vi "TCP_out_MSG.vi"(9 "msgin":string="MSGin") -> (1 "msg":string)   [LabVIEW 2019, in "FINS TCP.lvlib"]
uses:
  FINS TCP.lvlib
panel:
  out "length":u32
  # "FINS"
  # "Length"
  # "CMD"
  # "Error"
  # "Client Node"
  # "Server Node"
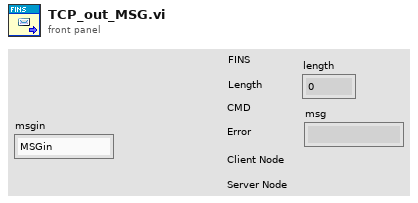
[diagram p1: front panel]
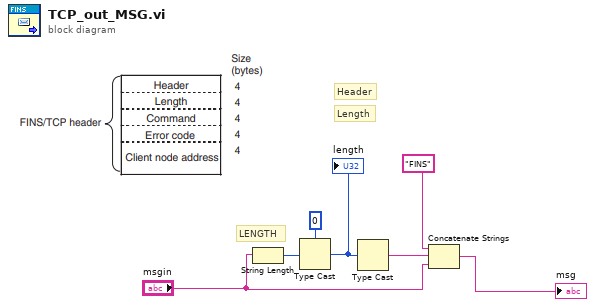
[diagram p0: block diagram]
diagram:
  # "Length"
  # "Header"
  # "LENGTH"
  n1 = String Length(string="msgin") -> (length=w1:i32)
  n2 = Type Cast(type=u32 0 ("length"), x=w1) -> (*(type *) &x=w6:u32)
  "length" <- w6
  n3 = Type Cast(x=w6) -> (*(type *) &x=w5:string)  [unwired: 1 in]
  n4 = Concatenate Strings("FINS" ("header"), w5, "msgin") -> (→"msg":string)
